vi "StressDist_shear_calc.vi"(1 "Angle":dbl, 2 "Parameters":dbl[](array[numeric])) -> (0 "Stress":dbl)   [LabVIEW 2016]
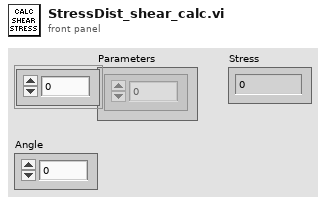
[diagram p1: front panel]
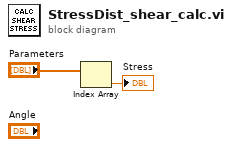
[diagram p0: block diagram]
diagram:
  n1 = Index Array(array="Parameters") -> (element=→"Stress":dbl)  [unwired: 1 in]
